vi "AccelerometerAccelerationCalculationLoop.vi"   [LabVIEW 2016]
uses:
  <vilib>/rvi/DataTransferAndStorage/Container/XNode/niFpgaContainer.xnode
  <userlib>/_NI FLP Library/FPGA/outsideSCTL/FlpLib Multiply Shared Instance 0.vi
  <vilib>/rvi/FIFO/Fifo_Resource/nirvififoEmulationRead.vi
  <vilib>/rvi/FIFO/Fifo_Resource/nirvififoEmulationWrite.vi
types:
  T1 = cluster{"Sample":u64, "Timestamp":u64, "Raw1":sgl, "Raw2":sgl, "Raw3":sgl, "Raw4":sgl, "Raw5":sgl, "Raw6":sgl, "Raw7":sgl, "Raw8":sgl}
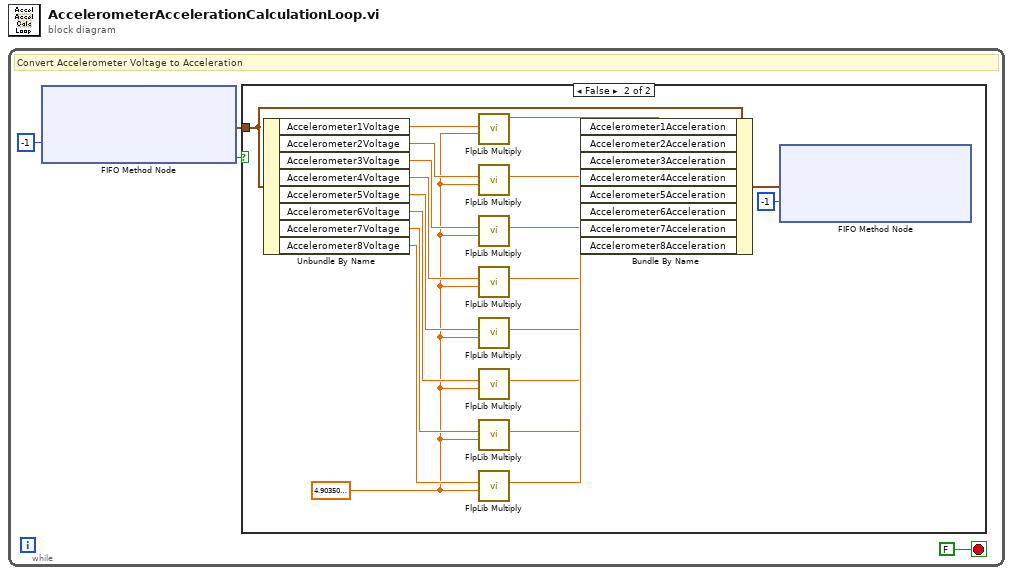
[diagram p0: block diagram]
diagram:
  n1 = while {
    stop <- FALSE stop-if-true
    # "Convert Accelerometer Voltage to Acceleration"
    n2 = xnode ("FIFO Method Node")("Timeout"=-1) -> ("Element"=w1:T1, "Timed Out?"=w3:bool)  [unwired: 1 in, 1 out]
    n3 = case shown="False" w3 {
      tunnel: w1 -> [_ w14]
      frame True {
      }
      frame False {
        w15 = sgl 4.9035 ("y")
        n4 = Unbundle By Name(w14) -> ("Accelerometer1Voltage"=w23:sgl, "Accelerometer2Voltage"=w16:sgl, "Accelerometer3Voltage"=w17:sgl, "Accelerometer4Voltage"=w18:sgl, "Accelerometer5Voltage"=w19:sgl, "Accelerometer6Voltage"=w20:sgl, "Accelerometer7Voltage"=w21:sgl, "Accelerometer8Voltage"=w22:sgl)
        n5 = call-poly <userlib>:"FlpLib Multiply.vi"("y"=w15, "x"=w23) -> ("x*y"=w12:sgl)  [unwired: 5 in]
        n6 = call-poly <userlib>:"FlpLib Multiply.vi"("y"=w15, "x"=w16) -> ("x*y"=w5:sgl)  [unwired: 5 in]
        n7 = call-poly <userlib>:"FlpLib Multiply.vi"("y"=w15, "x"=w17) -> ("x*y"=w6:sgl)  [unwired: 5 in]
        n8 = call-poly <userlib>:"FlpLib Multiply.vi"("y"=w15, "x"=w18) -> ("x*y"=w7:sgl)  [unwired: 5 in]
        n9 = call-poly <userlib>:"FlpLib Multiply.vi"("y"=w15, "x"=w19) -> ("x*y"=w8:sgl)  [unwired: 5 in]
        n10 = call-poly <userlib>:"FlpLib Multiply.vi"("y"=w15, "x"=w20) -> ("x*y"=w9:sgl)  [unwired: 5 in]
        n11 = call-poly <userlib>:"FlpLib Multiply.vi"("y"=w15, "x"=w21) -> ("x*y"=w10:sgl)  [unwired: 5 in]
        n12 = call-poly <userlib>:"FlpLib Multiply.vi"("y"=w15, "x"=w22) -> ("x*y"=w11:sgl)  [unwired: 5 in]
        n13 = Bundle By Name(cluster=w14, "Accelerometer1Acceleration"=w12, "Accelerometer2Acceleration"=w5, "Accelerometer3Acceleration"=w6, "Accelerometer4Acceleration"=w7, "Accelerometer5Acceleration"=w8, "Accelerometer6Acceleration"=w9, "Accelerometer7Acceleration"=w10, "Accelerometer8Acceleration"=w11) -> (w13:T1)
        n14 = xnode ("FIFO Method Node")("Element"=w13, "Timeout"=-1) -> ()  [unwired: 1 in, 2 out]
      }
    }
  }
